vi "Latch.vi"(1 "Input":bool) -> (0 "Output":bool)   [LabVIEW 2014]
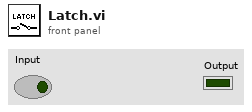
[diagram p1: front panel]
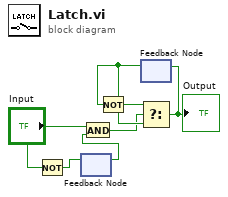
[diagram p0: block diagram]
diagram:
  n1 = Not(x="Input") -> (.not. x?=w5:bool)
  n2 = feedback-in #1(w5) -> ()
  n3 = feedback #1() -> (w4:bool)  [unwired: 1 in]
  n4 = And(x="Input", y=w4) -> (x .and. y?=w1:bool)
  n5 = feedback #2() -> (w2:bool)  [unwired: 1 in]
  n6 = Not(x=w2) -> (.not. x?=w7:bool)
  n7 = Select(t=w7, s=w1, f=w2) -> (s? t:f=w6:bool)
  "Output" <- w6
  n8 = feedback-in #2(w6) -> ()
